vi "Wing.vi"() -> ()   [LabVIEW 2017]
doc: "This example performs writes and reads on a serial port, as directed by the user. You can press the Write and Read buttons, and change the Read Count, while the example is running.\n\nThe parameters set for the serial port must match the parameters of the connected instrument or device. In this example, the Read Count parameter specifies the number of bytes that the serial port reads. If there were more bytes at the port than the specified number, those bytes would not be read. If there were less bytes at the port than the specified number, you would receive a timeout error.\n\nThis example expands upon the flow control options for XON and XOFF, allowing the user to choose those control characters. Also, the user can enable or disable a termination character. Some devices require a termination character in order to identify the end of command strings. Some devices send a termination character to signify the end of data to be read. This example shows how you can end the Read operation once a termination character is detected in the buffer and/or append a termination character at the end of the Write data."
uses:
  subVIs/Serial - Settings.ctl
  subVIs/Serial - XON-XOFF Characters.ctl
  subVIs/Serial - ASCII Characters.ctl
  <vilib>/Analysis/baseanly.llb/Mean (DBL).vi
  <vilib>/DAQmx/read.llb/DAQmx Read (Analog 2D DBL NChan NSamp).vi
  <vilib>/Analysis/baseanly.llb/A x Vector.vi
  <vilib>/Instr/_visa.llb/VISA Configure Serial Port (Instr).vi
  <vilib>/DAQmx/create/channels.llb/DAQmx Create Channel (AI-Voltage-Basic).vi
  <vilib>/DAQmx/configure/timing.llb/DAQmx Timing (Sample Clock).vi
  <vilib>/express/express shared/transition.llb/Dynamic To Waveform Array.vi
  <vilib>/express/express arith-compare/Formula/Block/exnFormulaBlock how many pts in the wave.vi
  <vilib>/express/express shared/ex_Modify Signal Name.vi
  <vilib>/express/express shared/transition.llb/Waveform Array To Dynamic.vi
  <vilib>/DAQmx/miscellaneous.llb/DAQmx Fill In Error Info.vi
  <vilib>/express/express signal manip/GetorSetDDTAttributes/Set DDT Attributes/SetT0.vi
  <vilib>/express/express arith-compare/Formula/XNode/ExpressFormulaBlockNode.xnode
  <vilib>/express/express signal manip/GetorSetDDTAttributes/Set DDT Attributes/Set DDT Properties.xnode
  <vilib>/regexp/Match Regular Expression.xnode
  <vilib>/Analysis/NI_AALBase.lvlib
panel:
  out "New Bias Volt":dbl[][](array[numeric])
  out "New Bias Vec":dbl[](array[numeric])
  in  "Transform":T1
  in  "Tab Control":T2(tab)
  out "Drag (N)":dbl format="%#_3g"
  out "Lift (N)":dbl format="%#_3g"
  out "Calculated Density":dbl
  in  "Specific Gas Constant R":dbl
  in  "Ambient Temperature":dbl
  in  "Ambient Pressure":dbl
  out "Raw Voltage":dbl format="%#_4g"
  out "Airspeed":dbl
  out "Dynamic Pressure":dbl format="%#_4g"
  out "Transformed Lift and Drag Data":cluster{dbl, dbl}(graph)
  out "Position\n(relative to zeroed position)":dbl format="%#.3g"
  in  "Initiate Traverse&Log":bool
  in  "Stepper Control COM Port\n(changes require VI restart)":refnum<visa-resource-name>="COM1"
  out "Motion Status":string
  out "Controller Time":string
  out "Torque Units 2":string
  out "Force Units 2":string
  out "Measurement":dbl[][](graph) caption="Resolved Load Cell Data"
  in  "Bias":bool
  in  "Unbias":bool
  in  "Traverse Sweep":bool
  in  "Jog":bool
  in  "Jog Step (deg)":dbl
  in  "Zero":bool
  in  "Go Home":bool
  in  "Stop Motor":bool
  in  "Jog Mode":bool
  in  "1°":bool
  in  "0.25°":bool
  in  "-0.25°":bool
  in  "-1°":bool
  out "Factory-Calculated Calibration Matrix":dbl[][](array[numeric])
  out "Raw Strain Gauge Voltages":dbl[][](array[numeric]) format="%#_4g"
  out "Forces/Torques (X Y Z L M N) (N/Nm)":dbl[][](array[numeric]) format="%0.2f"
  out "Biased Voltages":dbl[](array[numeric]) format="%#.4g"
  out "RegEx 3":string
  out "whole match 3":string
  out "RegEx 2":string
  out "whole match 2":string
  out "whole match":string
  out "RegEx":string
  # "Data Collection"
  # "Wing Position Control"
  # "deg"
  # "Wind Speed Using Baratron"
  # "Air Density Calculation"
  # "1.016mmHg = 1 V"
  # "kPa"
  # "J/kgK"
  # "kg/m^3"
  # "C"
  # "Torr"
  # "m/s"
  # "Voltage to Load Conversions"
  # "-"
  # "="
  # "("
  # ")"
  # "x"
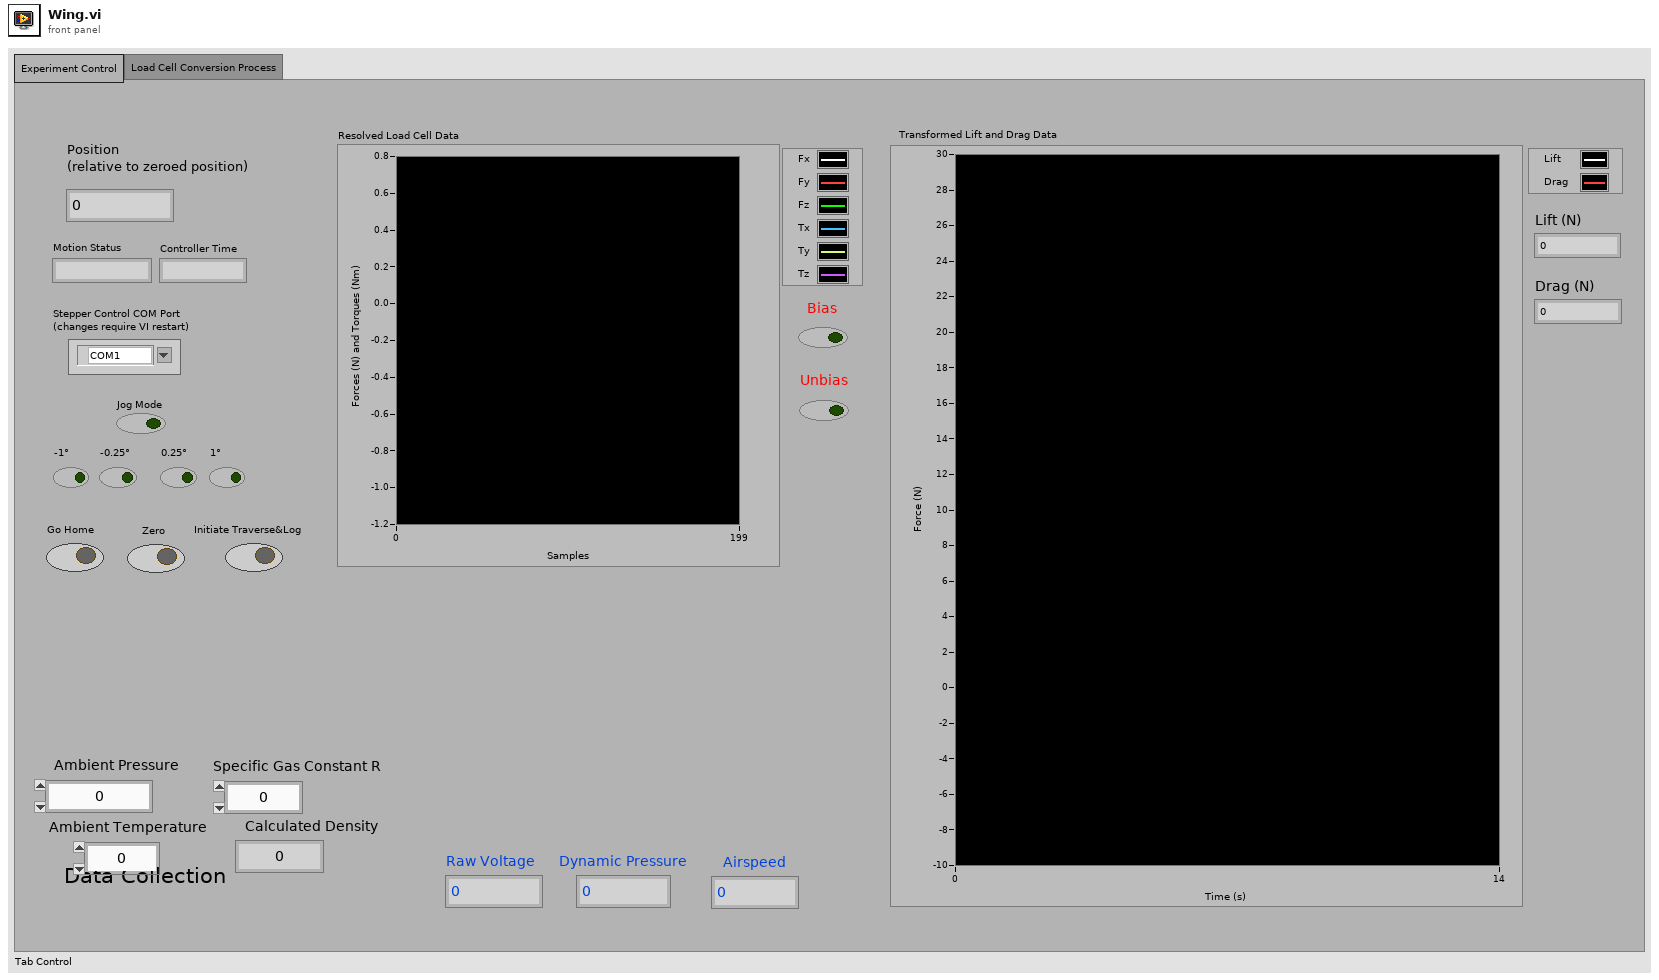
[diagram p1: front panel]
types:
  T1 = cluster{"Dx":dbl, "Dy":dbl, "Dz":dbl, "Rx":dbl, "Ry":dbl, "Rz":dbl}
  T2 = enum32{"Experiment Control", "Load Cell Conversion Process"}
  T3 = typedef "Serial - XON-XOFF Characters.ctl" = cluster{"XON":T4, "XOFF":T4}
  T4 = typedef "Serial - ASCII Characters.ctl" = enum16{"NUL", "SOH", "STX", "ETX", "EOT", "ENQ", "ACK", "BEL", "BS", "HT", "LF", "VT", "FF", "CR", "SO", "SI", "DLE", "DC1", "DC2", "DC3", "DC4", "NAK", "SYN", "ETB", "CAN", "EM", "SUB", "ESC", "FS", "GS", "RS", "US", "SP", "!", "\"", "#", "$", "%", "&", "'", "(", ")", "*", "+", ",", "- (-)", ".", "/", "0", "1", "2", "3", "4", "5", "6", "7", "8", "9", ":", ";", "<", "=", ">", "?", "@", "A", "B", "C", "D", "E", "F", "G", "H", "I", "J", "K", "L", "M", "N", "O", "P", "Q", "R", "S", "T", "U", "V", "W", "X", "Y", "Z", "[", "\\", "]", "^", "_", "`", "a", "b", "c", "d", "e", "f", "g", "h", "i", "j", "k", "l", "m", "n", "o", "p", "q", "r", "s", "t", "u", "v", "w", "x", "y", "z", "{", "|", "}", "~"}
  T5 = typedef "Serial - Settings.ctl" = cluster{"baud rate":u32, "data bits":u16, "parity":enum16{"None", "Odd", "Even", "Mark", "Space"}, "stop bits":u16, "flow control":u16}
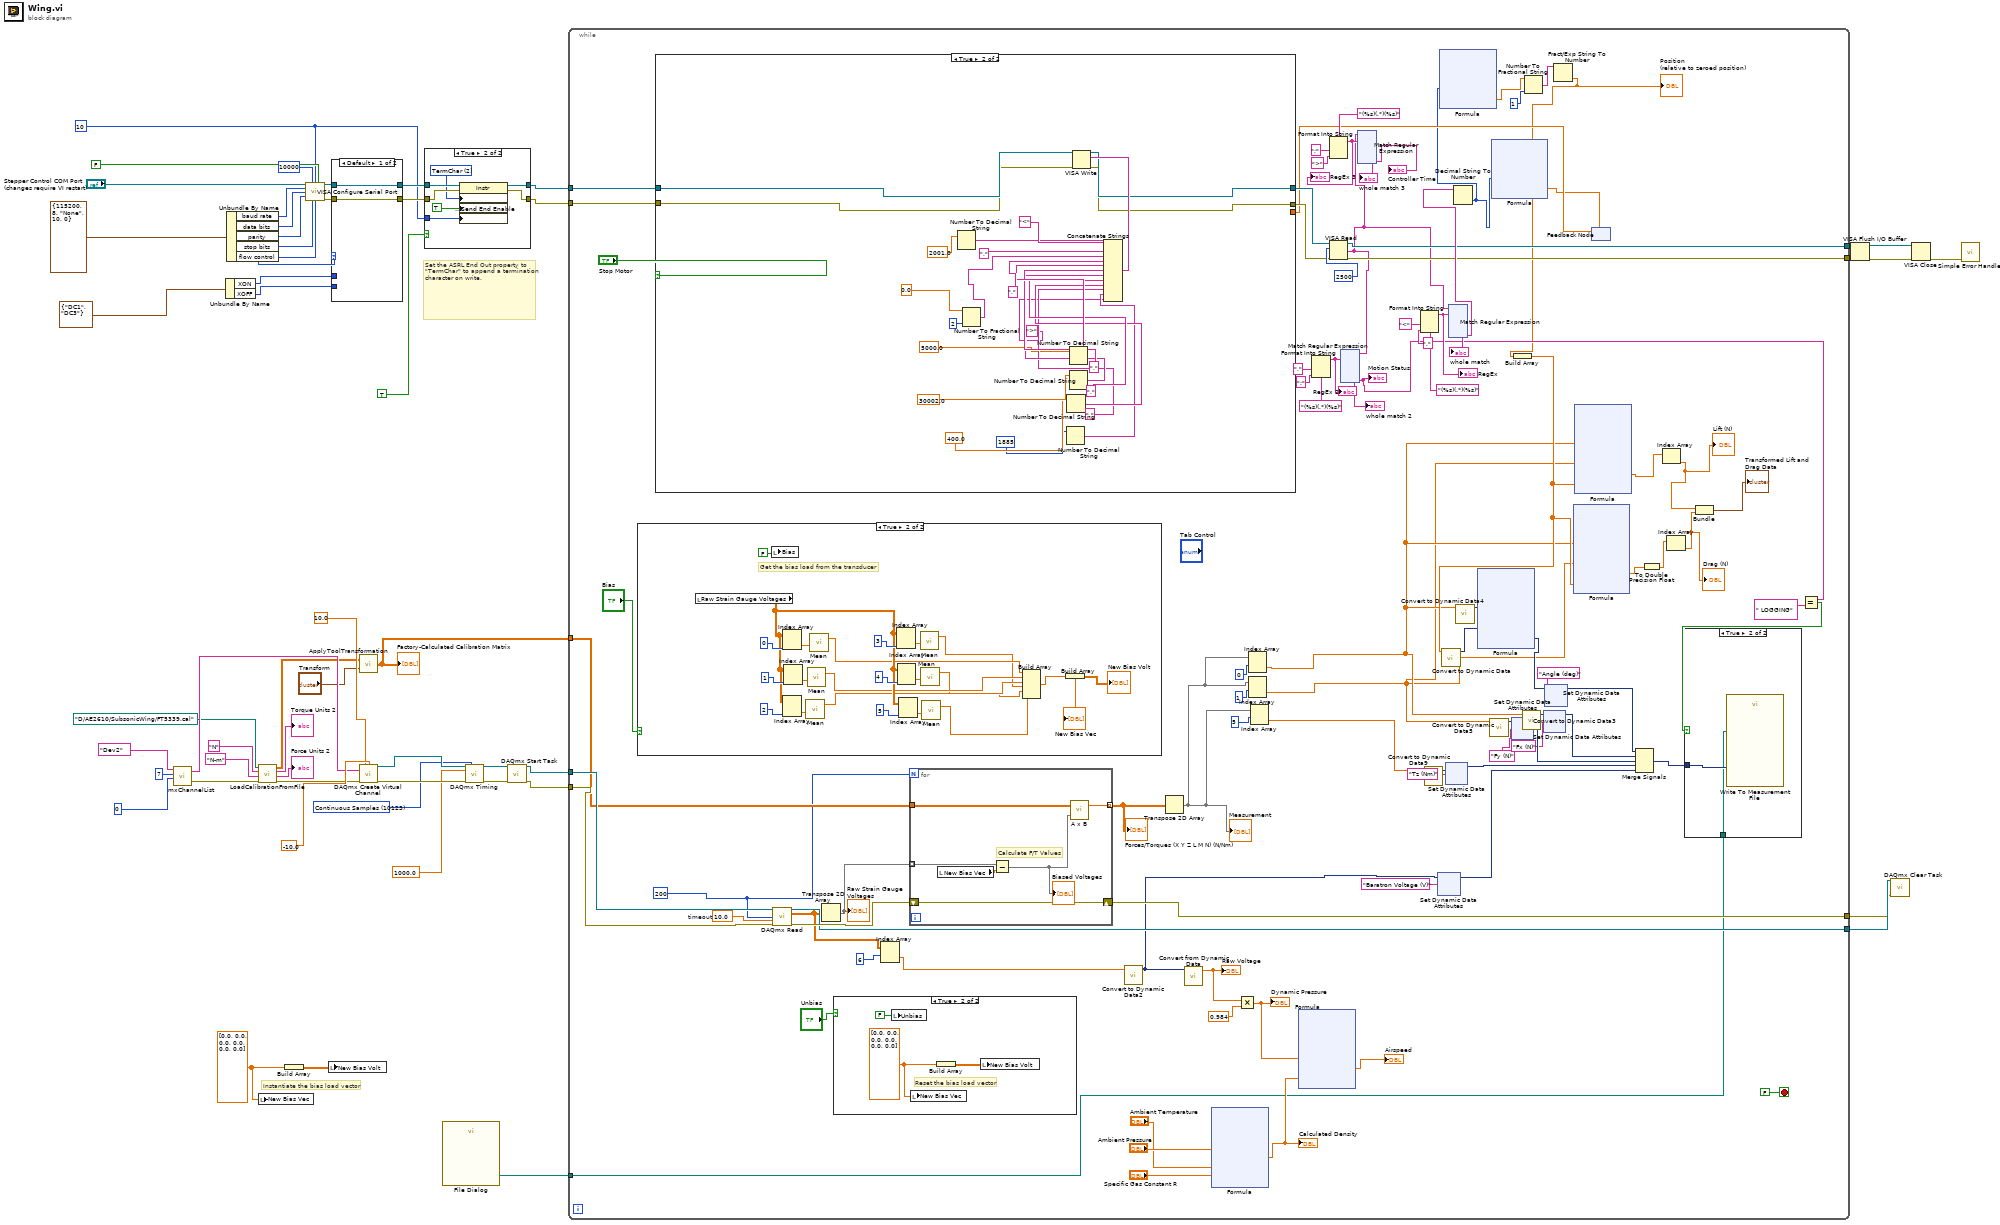
[diagram p0: block diagram]
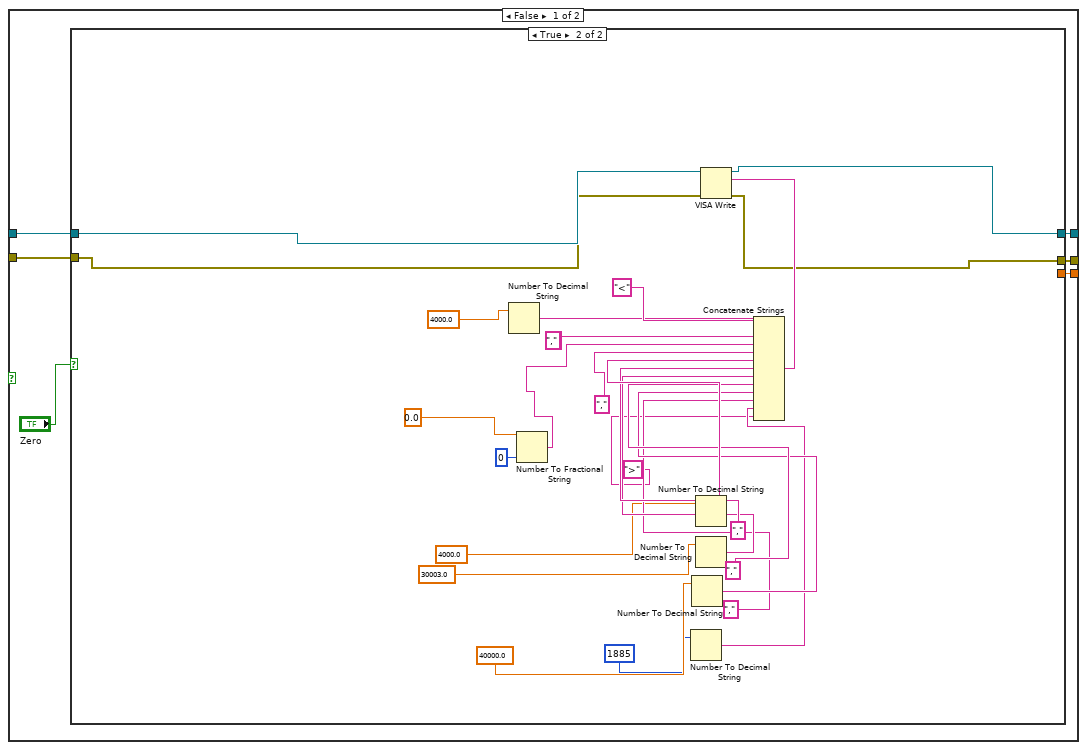
[diagram p5: hidden frame]
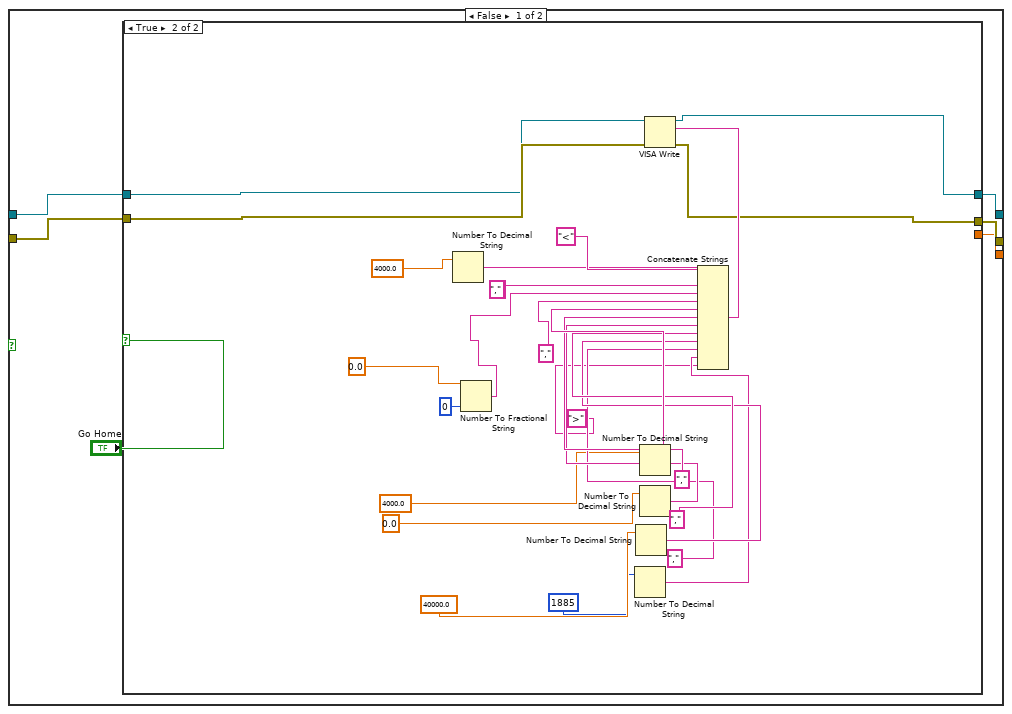
[diagram p6: hidden frame]
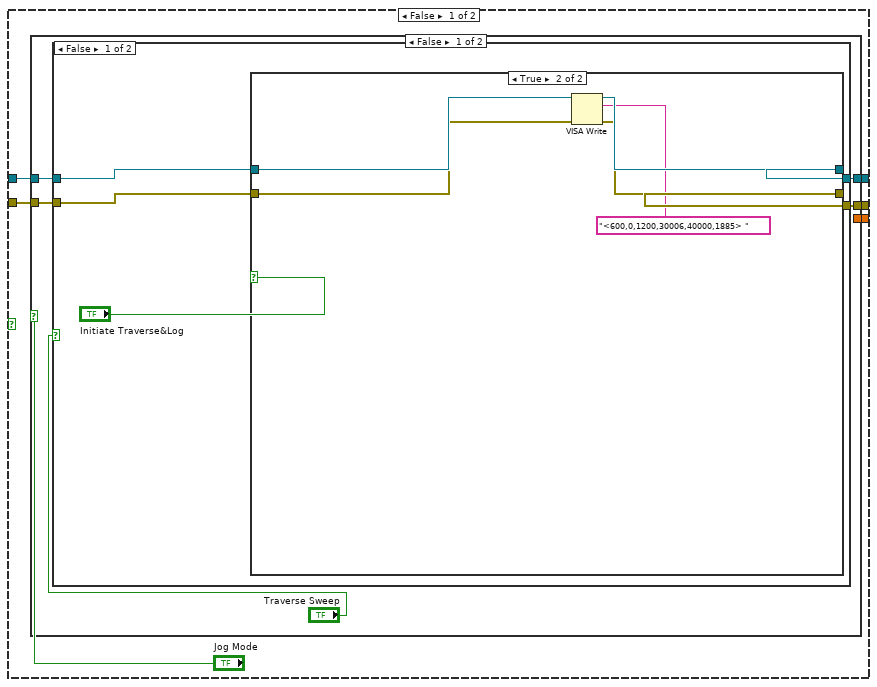
[diagram p7: hidden frame]
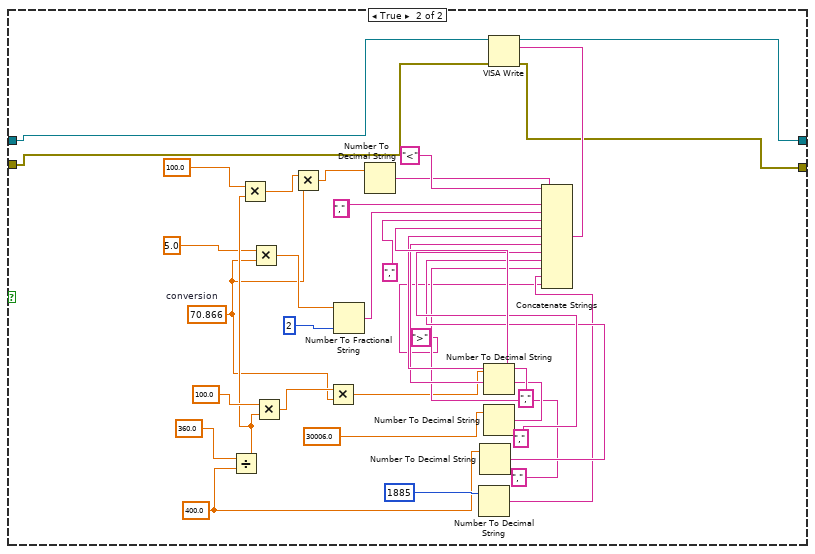
[diagram p9: hidden frame]
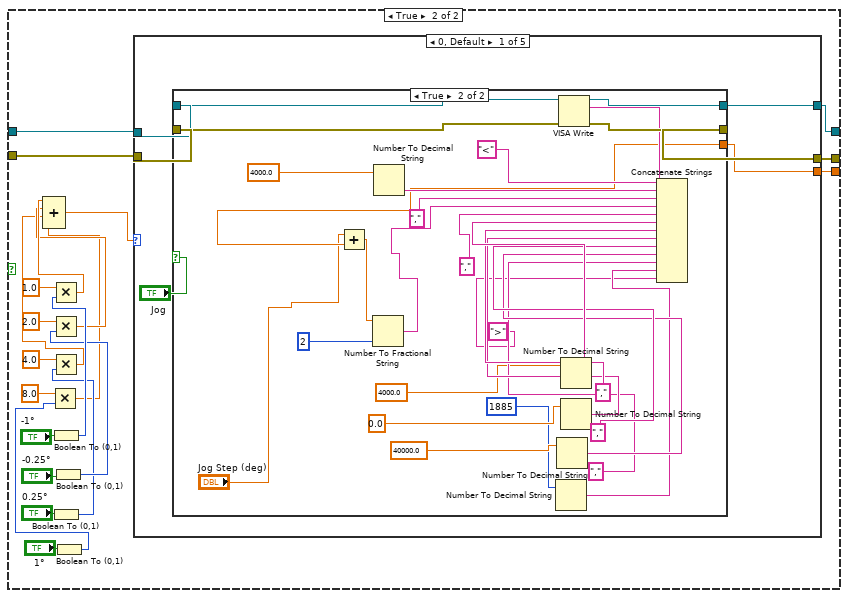
[diagram p10: hidden frame]
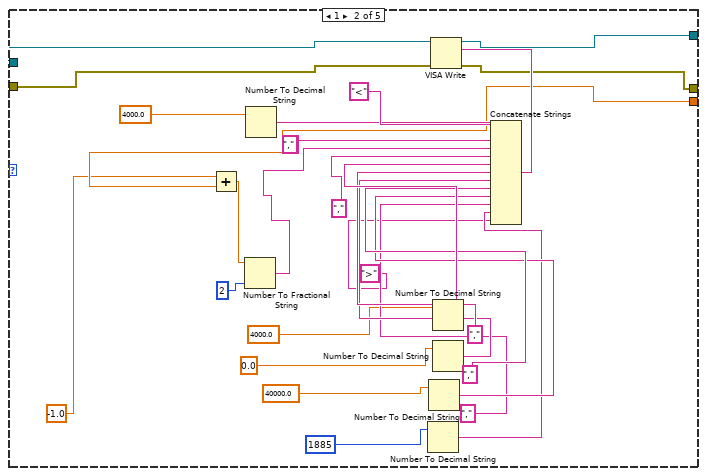
[diagram p12: hidden frame]
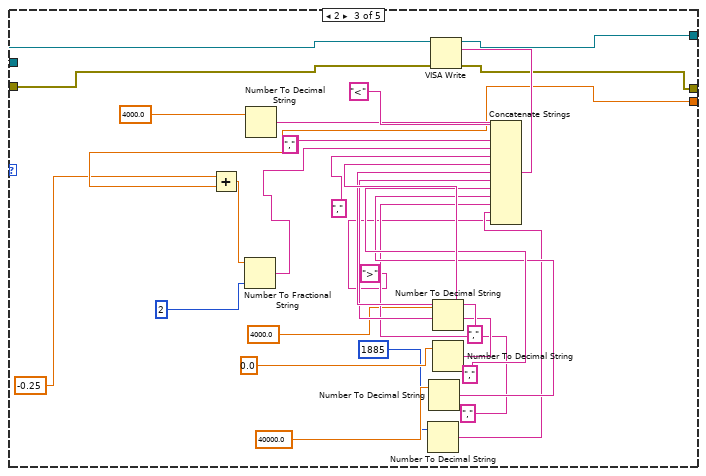
[diagram p13: hidden frame]
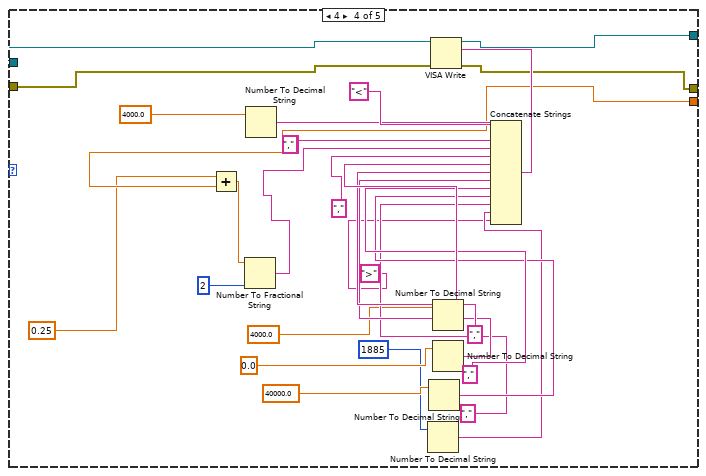
[diagram p14: hidden frame]
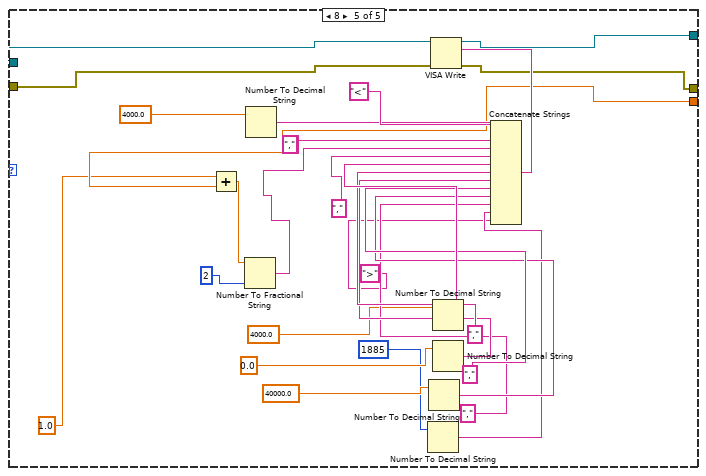
[diagram p15: hidden frame]
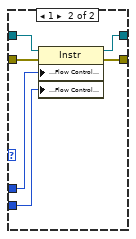
[diagram p17: hidden frame]
diagram:
  w2 = dbl[] [0.0, 0.0, 0.0, 0.0, 0.0, 0.0]
  w25 = 10123 items=["Finite Samples"=10178, "Continuous Samples"=10123] ("sample mode")
  w37 = u8 10 ("Termination Character")
  # "Instantiate the bias load vector"
  # "Set the ASRL End Out property to \"TermChar\" to append a termination character on write."
  n1 = call "mxChannelList.vi"("First Channel"=i16 0, "Number of Channels"=7, "DAQmx Device Name"=tag "Dev2" ("DAQ Card")) -> ("error out"=w10:errorcluster, "Channel List"=w19:string)  [unwired: 1 in]
  n2 = Unbundle By Name(T3 {"XON"=enum."DC1", "XOFF"=enum."DC3"} ("XON/XOFF Characters")) -> ("XON"=w42:T4, "XOFF"=w41:T4)
  n3 = Unbundle By Name(T5 {"baud rate"=115200, "data bits"=8, "parity"=enum."None", "stop bits"=10, "flow control"=0} ("Serial Settings")) -> ("baud rate"=w47:u32, "data bits"=w48:u16, "parity"=w49:enum16{"None", "Odd", "Even", "Mark", "Space"}, "stop bits"=w50:u16, "flow control"=w43:u16)
  n4 = call "LoadCalibrationFromFile.vi"("Error In"=w10, "User Torque Units"="N-m" ("Torque Units"), "User Force Units"="N" ("Force Units"), "Cal File Path"=path "D:/AE2610/SubsonicWing/FT5339.cal" ("Calibration File")) -> ("Error Out"=w9:errorcluster, "Calibration Force Units"=→"Force Units 2":string, "Calibration Torque Units"=→"Torque Units 2":string, "Calibration Matrix"=w15:dbl[][])
  n5 = local write "New Bias Vec"(w2) -> ()
  n6 = Build Array(w2) -> (w1:dbl[][])
  n7 = call-poly "VISA Configure Serial Port"("VISA resource name"="Stepper Control COM Port\n(changes require VI restart)", "timeout (10sec)"=u32 10000, "termination char\n(0xA = '\\n' = LF)"=w37, "Enable Termination\nChar (T)"=FALSE ("End Read on Termination Character?"), "baud rate (9600)"=w47, "data bits (8)"=w48, "parity (0:none)"=w49, "stop bits (10: 1 bit)"=w50, "flow control (0:none)"=w43) -> ("VISA resource name out"=w51:refnum<visa-resource-name>, "error out"=w52:errorcluster)  [unwired: 1 in, 4 out]
  n8 = local write "New Bias Volt"(w1) -> ()
  n9 = case shown="Default" w43 {
    tunnel: [w55 w62] -> w40
    tunnel: [w56 w61] -> w39
    tunnel: w52 -> [w55 w60]
    tunnel: w51 -> [w56 w59]
    tunnel: w42 -> [_ w58]
    tunnel: w41 -> [_ w57]
    frame Default {
    }
    frame 1 {
      n10 = property class="Instr"(reference=w59, error in=w60, "Serial Settings:Flow Control XON Character"=w58, "Serial Settings:Flow Control XOFF Character"=w57) -> (reference out=w61:refnum<visa-resource-name>, error out=w62:errorcluster)
    }
  }
  n11 = call "ApplyToolTransformation.vi"("Transform"="Transform", "Calibration Matrix"=w15) -> ("Transformed Calibration Matrix"=w6:dbl[][])
  "Factory-Calculated Calibration Matrix" <- w6
  n12 = call-poly <vilib>:"DAQmx Create Virtual Channel.vi"("maximum value"=10.0 ("Maximum Value"), "minimum value"=-10.0 ("Minimum Value"), "physical channels"=w19, "error in"=w9) -> ("task out"=w26:refnum<k21>, "error out"=w27:errorcluster)  [unwired: 10 in]
  n13 = case shown="True" TRUE ("End Write on Termination Character?") {
    tunnel: w39 -> [w63 w71]
    tunnel: w40 -> [w64 w70]
    tunnel: [w63 w69] -> w36
    tunnel: [w64 w68] -> w35
    tunnel: w37 -> [_ w66]
    frame False {
    }
    frame True {
      w67 = u16 2 items=["None", "LastBit", "TermChar", "Break"] ("Serial Settings:Serial End Mode for Writes")
      n14 = property class="Instr"(reference=w71, error in=w70, "Serial Settings:End Mode for Writes"=w67, "Message Based Settings:Send End Enable"=TRUE, "Message Based Settings:Termination Character"=w66) -> (reference out=w69:refnum<visa-resource-name>, error out=w68:errorcluster)
    }
  }
  n15 = call "File Dialog"() -> ("selected path"=w3:path)  [unwired: 12 in, 3 out]
  n16 = call-poly <vilib>:"DAQmx Timing.vi"("task/channels in"=w26, "sample mode"=w25, "rate"=1000.0 ("Sample Rate"), "error in"=w27) -> ("task out"=w24:refnum<k21>, "error out"=w18:errorcluster)  [unwired: 10 in]
  n17 = call <vilib>:"DAQmx Start Task.vi"("task/channels in"=w24, "error in"=w18) -> ("task out"=w8:refnum<k21>, "error out"=w7:errorcluster)  [unwired: 12 in]
  n18 = while {
    tunnel: w36 -> [w149]
    tunnel: w35 -> [w148]
    tunnel: [w147] -> w33
    tunnel: [w146] -> w34
    tunnel: w8 -> [w133]
    tunnel: w7 -> [w132]
    tunnel: w6 -> [w129]
    tunnel: [w127] -> w5
    tunnel: [w124] -> w4
    tunnel: w3 -> [w85]
    stop <- FALSE stop-if-true
    w128 = 200 ("Samples to Read")
    w134 = 10.0  # timeout
    n19 = case shown="True" "Bias" {
      frame False {
      }
      frame True {
        # "Get the bias load from the transducer"
        n20 = local read "Raw Strain Gauge Voltages"() -> (w705:dbl[][])
        n21 = local write "Bias"(FALSE) -> ()
        n22 = Index Array(array=w705, index (col)=0 ("disabled index (col)")) -> (element=w718:dbl[])  [unwired: 1 in]
        n23 = Index Array(array=w705, index (col)=2 ("disabled index (col)")) -> (element=w713:dbl[])  [unwired: 1 in]
        n24 = Index Array(array=w705, index (col)=1 ("disabled index (col)")) -> (element=w715:dbl[])  [unwired: 1 in]
        n25 = call-poly <vilib>:"Mean.vi"("X"=w713) -> ("mean"=w702:dbl)  [unwired: 1 out]
        n26 = call-poly <vilib>:"Mean.vi"("X"=w715) -> ("mean"=w703:dbl)  [unwired: 1 out]
        n27 = call-poly <vilib>:"Mean.vi"("X"=w718) -> ("mean"=w704:dbl)  [unwired: 1 out]
        n28 = Index Array(array=w705, index (col)=3 ("disabled index (col)")) -> (element=w711:dbl[])  [unwired: 1 in]
        n29 = Index Array(array=w705, index (col)=4 ("disabled index (col)")) -> (element=w709:dbl[])  [unwired: 1 in]
        n30 = Index Array(array=w705, index (col)=5 ("disabled index (col)")) -> (element=w707:dbl[])  [unwired: 1 in]
        n31 = call-poly <vilib>:"Mean.vi"("X"=w711) -> ("mean"=w701:dbl)  [unwired: 1 out]
        n32 = call-poly <vilib>:"Mean.vi"("X"=w709) -> ("mean"=w700:dbl)  [unwired: 1 out]
        n33 = call-poly <vilib>:"Mean.vi"("X"=w707) -> ("mean"=w699:dbl)  [unwired: 1 out]
        n34 = Build Array(w704, w703, w702, w701, w700, w699) -> (w698:dbl[])
        "New Bias Vec" <- w698
        n35 = Build Array(w698) -> (→"New Bias Volt":dbl[][])
      }
    }
    n36 = call-poly <vilib>:"DAQmx Read.vi"("task/channels in"=w133, "number of samples per channel"=w128, "timeout"=w134, "error in"=w132) -> ("task out"=w127:refnum<k21>, "data"=w96:dbl[][], "error out"=w131:errorcluster)  [unwired: 9 in]
    n37 = Transpose 2D Array(2D array=w96) -> (transposed array=w130:dbl[][])
    "Raw Strain Gauge Voltages" <- w130
    n38 = case shown="True" "Unbias" {
      frame False {
      }
      frame True {
        w695 = dbl[] [0.0, 0.0, 0.0, 0.0, 0.0, 0.0]
        # "Reset the bias load vector"
        n39 = local write "Unbias"(FALSE) -> ()
        n40 = local write "New Bias Vec"(w695) -> ()
        n41 = Build Array(w695) -> (w694:dbl[][])
        n42 = local write "New Bias Volt"(w694) -> ()
      }
    }
    n43 = Index Array(array=w96, index (row)=6) -> (element=w94:dbl[])  [unwired: 1 in]
    n44 = for {
      N: w128 -> [_]
      tunnel: [w722] -> w120 mode=indexing
      shift-right: [w721] -> w124
      shift-left: w131 -> [w721]
      tunnel: w130 -> [w724] mode=indexing
      tunnel: w129 -> [w720]
      # "Calculate F/T Values"
      n45 = local read "New Bias Vec"() -> (w723:dbl[])
      n46 = Subtract(x=w724, y=w723) -> (x-y=w719:dbl[])
      "Biased Voltages" <- w719
      n47 = call-poly <vilib>:"A x B.vi"("Vector"=w719, "A"=w720) -> ("A x Vector"=w722:dbl[])  [unwired: 1 out]
    }
    "Forces/Torques (X Y Z L M N) (N/Nm)" <- w120
    n48 = call "Convert to Dynamic Data2"("Array"=w94) -> ("Dynamic Data Type"=w76:dynamicdata)  [unwired: 3 in]
    n49 = Transpose 2D Array(2D array=w120) -> (transposed array=w119:dbl[][])
    "Measurement" <- w119
    n50 = call "Convert from Dynamic Data"("Dynamic Data Type"=w76) -> ("Scalar"=w91:dbl)  [unwired: 3 in]
    "Raw Voltage" <- w91
    n51 = xnode "Formula"("P"="Ambient Pressure", "T"="Ambient Temperature", "R"="Specific Gas Constant R") -> ("Result"=w87:dbl)  [unwired: 1 in, 1 out]
    "Calculated Density" <- w87
    n52 = Multiply(x=w91, y=0.984) -> (x*y=w84:dbl)
    "Dynamic Pressure" <- w84
    n53 = Index Array(array=w119, index (row)=0 ("index")) -> (element=w83:dbl[])  [unwired: 1 in]
    n54 = Index Array(array=w119, index (row)=1 ("index")) -> (element=w80:dbl[])  [unwired: 1 in]
    n55 = Index Array(array=w119, index (row)=5 ("index")) -> (element=w78:dbl[])  [unwired: 1 in]
    n56 = xnode "Formula"("del P"=w84, "Density"=w87) -> ("Result"=→"Airspeed":dbl)  [unwired: 1 in, 1 out]
    n57 = Format Into String(format string="(%s)(.*)(%s)", "," ("WordBefore"), ";" ("WordAfter")) -> (resulting string=w163:string)  [unwired: 2 in, 1 out]
    "RegEx 2" <- w163
    n58 = Format Into String(format string="(%s)(.*)(%s)", ";" ("WordBefore"), ">" ("WordAfter")) -> (resulting string=w145:string)  [unwired: 2 in, 1 out]
    "RegEx 3" <- w145
    n59 = Format Into String(format string="(%s)(.*)(%s)", "<" ("WordBefore"), "," ("WordAfter")) -> (resulting string=w160:string)  [unwired: 2 in, 1 out]
    "RegEx" <- w160
    n60 = call "Convert to Dynamic Data9"("Array"=w78) -> ("Dynamic Data Type"=w77:dynamicdata)  [unwired: 3 in]
    n61 = xnode ("Set Dynamic Data Attributes")("Signals In"=w76, "Signal Name"="Baratron Voltage (V)") -> ("Signals Out"=w74:dynamicdata)  [unwired: 2 in, 1 out]
    n62 = xnode ("Set Dynamic Data Attributes")("Signals In"=w77, "Signal Name"="Tz (Nm)") -> ("Signals Out"=w75:dynamicdata)  [unwired: 2 in, 1 out]
    n63 = call "Convert to Dynamic Data4"("Array"=w83) -> ("Dynamic Data Type"=w81:dynamicdata)  [unwired: 3 in]
    n64 = call "Convert to Dynamic Data5"("Array"=w80) -> ("Dynamic Data Type"=w79:dynamicdata)  [unwired: 3 in]
    n65 = xnode ("Set Dynamic Data Attributes")("Signals In"=w79, "Signal Name"="Fy (N)") -> ("Signals Out"=w114:dynamicdata)  [unwired: 2 in, 1 out]
    n66 = call "Convert to Dynamic Data3"("Array"=w83) -> ("Dynamic Data Type"=w82:dynamicdata)  [unwired: 3 in]
    n67 = xnode ("Set Dynamic Data Attributes")("Signals In"=w82, "Signal Name"="Fx (N)") -> ("Signals Out"=w115:dynamicdata)  [unwired: 2 in, 1 out]
    n68 = feedback #1() -> (w137:dbl)  [unwired: 1 in]
    n69 = case shown="True" "Stop Motor" {
      tunnel: [w738 w1016] -> w157
      tunnel: [w737 w1017] -> w156
      tunnel: w149 -> [w736 w1019]
      tunnel: w148 -> [w735 w1018]
      tunnel: w137 -> [w734 _]
      frame False {
        n70 = case shown="True" "Zero" {
          tunnel: [w744 w991] -> w738
          tunnel: [w743 w992] -> w737
          tunnel: w736 -> [w742 w994]
          tunnel: w735 -> [w741 w993]
          tunnel: w734 -> [w740 _]
          frame False {
            n71 = case shown="True" "Go Home" {
              tunnel: [w750 w966] -> w744
              tunnel: [w749 w967] -> w743
              tunnel: w742 -> [w748 w968]
              tunnel: w741 -> [w747 w969]
              tunnel: w740 -> [w745 _]
              frame False {
                n72 = case shown="False" "Jog Mode" {
                  tunnel: [w755 w818] -> w750
                  tunnel: [w754 w819] -> w749
                  tunnel: w748 -> [w753 w822]
                  tunnel: w747 -> [w752 w821]
                  tunnel: w745 -> [_ w820]
                  frame False {
                    n73 = case shown="False" "Traverse Sweep" {
                      tunnel: [w759 w769] -> w755
                      tunnel: [w758 w768] -> w754
                      tunnel: w753 -> [w757 w771]
                      tunnel: w752 -> [w756 w770]
                      frame False {
                        n74 = case shown="True" "Initiate Traverse&Log" {
                          tunnel: w757 -> [w762 w767]
                          tunnel: w756 -> [w761 w766]
                          tunnel: [w762 w765] -> w758
                          tunnel: [w761 w764] -> w759
                          frame False {
                          }
                          frame True {
                            n75 = VISA Write(VISA resource name=w767, write buffer="<600,0,1200,30006,40000,1885> ", error in (no error)=w766) -> (VISA resource name out=w765:refnum<visa-resource-name>, error out=w764:errorcluster)  [unwired: 1 out]
                          }
                        }
                      }
                      frame True {
                        w783 = 400.0 ("Steps/rev 2")
                        w772 = 70.866  # conversion
                        (unwired) ","
                        n76 = Divide(x=360.0, y=w783) -> (x/y=w779:dbl)
                        n77 = Multiply(x=100.0 ("Acceleration (mm/s^2) 2"), y=w779) -> (x*y=w774:dbl)
                        n78 = Multiply(x=5.0 ("Position (mm) 2"), y=w772) -> (x*y=w778:dbl)
                        n79 = Multiply(x=100.0 ("Velocity (mm/s) 2"), y=w779) -> (x*y=w776:dbl)
                        n80 = Multiply(x=w774, y=w772) -> (x*y=w773:dbl)
                        n81 = Multiply(x=w776, y=w772) -> (x*y=w775:dbl)
                        n82 = Number To Fractional String(number=w778, precision (6)=i16 2) -> (F-format string=w785:string)  [unwired: 2 in]
                        n83 = Number To Decimal String(number=w773) -> (decimal integer string=w797:string)  [unwired: 1 in]
                        n84 = Number To Decimal String(number=1885 ("Password 2")) -> (decimal integer string=w788:string)  [unwired: 1 in]
                        n85 = Number To Decimal String(number=w783) -> (decimal integer string=w790:string)  [unwired: 1 in]
                        n86 = Number To Decimal String(number=w775) -> (decimal integer string=w794:string)  [unwired: 1 in]
                        n87 = Number To Decimal String(number=30006.0 ("Number of Bounces 2")) -> (decimal integer string=w792:string)  [unwired: 1 in]
                        n88 = Concatenate Strings("<", w797, ",", w785, ",", w794, ",", w792, ",", w790, ",", w788, ">") -> (w786:string)
                        n89 = VISA Write(VISA resource name=w771, write buffer=w786, error in (no error)=w770) -> (VISA resource name out=w768:refnum<visa-resource-name>, error out=w769:errorcluster)  [unwired: 1 out]
                      }
                    }
                  }
                  frame True {
                    n90 = Boolean To (0,1)(Boolean="-1°") -> (0, 1=w809:i16)
                    n91 = Multiply(x=1.0, y=w809) -> (x*y=w805:dbl)
                    n92 = Boolean To (0,1)(Boolean="0.25°") -> (0, 1=w807:i16)
                    n93 = Multiply(x=4.0, y=w807) -> (x*y=w803:dbl)
                    n94 = Boolean To (0,1)(Boolean="-0.25°") -> (0, 1=w808:i16)
                    n95 = Multiply(x=2.0, y=w808) -> (x*y=w804:dbl)
                    n96 = Boolean To (0,1)(Boolean="1°") -> (0, 1=w806:i16)
                    n97 = Multiply(x=8.0, y=w806) -> (x*y=w802:dbl)
                    n98 = Compound Arithmetic op=ADD(w805, w804, w803, w802) -> (w801:dbl)
                    n99 = case shown="0, Default" w801 {
                      tunnel: w822 -> [w826 w860 w888 w915 w942]
                      tunnel: w821 -> [w827 w861 w889 w916 w943]
                      tunnel: w820 -> [w823 w859 w887 w914 w941]
                      tunnel: [w825 w863 w891 w918 w945] -> w819
                      tunnel: [w824 w862 w890 w917 w944] -> w818
                      frame 0, Default {
                        n100 = case shown="True" "Jog" {
                          tunnel: w826 -> [w830 w857]
                          tunnel: w827 -> [w829 w856]
                          tunnel: [w830 w855] -> w825
                          tunnel: [w829 w854] -> w824
                          tunnel: w823 -> [_ w833]
                          frame False {
                          }
                          frame True {
                            n101 = Add(x="Jog Step (deg)", y=w833) -> (x+y=w832:dbl)
                            n102 = Number To Fractional String(number=w832, precision (6)=i16 2) -> (F-format string=w835:string)  [unwired: 2 in]
                            n103 = Number To Decimal String(number=4000.0 ("Acceleration (steps/s) 2")) -> (decimal integer string=w848:string)  [unwired: 1 in]
                            n104 = Number To Decimal String(number=1885 ("Password 2")) -> (decimal integer string=w839:string)  [unwired: 1 in]
                            n105 = Number To Decimal String(number=40000.0 ("Steps/rev 2")) -> (decimal integer string=w841:string)  [unwired: 1 in]
                            n106 = Number To Decimal String(number=4000.0 ("Velocity (steps/s) 2")) -> (decimal integer string=w845:string)  [unwired: 1 in]
                            n107 = Number To Decimal String(number=0.0 ("Number of Bounces 2")) -> (decimal integer string=w843:string)  [unwired: 1 in]
                            n108 = Concatenate Strings("<", w848, ",", w835, ",", w845, ",", w843, ",", w841, ",", w839, ">") -> (w837:string)
                            n109 = VISA Write(VISA resource name=w857, write buffer=w837, error in (no error)=w856) -> (VISA resource name out=w855:refnum<visa-resource-name>, error out=w854:errorcluster)  [unwired: 1 out]
                          }
                        }
                      }
                      frame 1 {
                        (unwired) ","
                        n110 = Add(x=-1.0 ("Jog Step (angle) 2"), y=w859) -> (x+y=w864:dbl)
                        n111 = Number To Fractional String(number=w864, precision (6)=i16 2) -> (F-format string=w866:string)  [unwired: 2 in]
                        n112 = Number To Decimal String(number=4000.0 ("Acceleration (steps/s) 2")) -> (decimal integer string=w879:string)  [unwired: 1 in]
                        n113 = Number To Decimal String(number=1885 ("Password 3")) -> (decimal integer string=w870:string)  [unwired: 1 in]
                        n114 = Number To Decimal String(number=40000.0 ("Steps/rev 3")) -> (decimal integer string=w872:string)  [unwired: 1 in]
                        n115 = Number To Decimal String(number=4000.0 ("Velocity (steps/s) 2")) -> (decimal integer string=w876:string)  [unwired: 1 in]
                        n116 = Number To Decimal String(number=0.0 ("Number of Bounces 2")) -> (decimal integer string=w874:string)  [unwired: 1 in]
                        n117 = Concatenate Strings("<", w879, ",", w866, ",", w876, ",", w874, ",", w872, ",", w870, ">") -> (w868:string)
                        n118 = VISA Write(VISA resource name=w860, write buffer=w868, error in (no error)=w861) -> (VISA resource name out=w863:refnum<visa-resource-name>, error out=w862:errorcluster)  [unwired: 1 out]
                      }
                      frame 2 {
                        (unwired) ","
                        n119 = Add(x=-0.25 ("Jog Step (angle) 2"), y=w887) -> (x+y=w892:dbl)
                        n120 = Number To Fractional String(number=w892, precision (6)=i16 2) -> (F-format string=w893:string)  [unwired: 2 in]
                        n121 = Number To Decimal String(number=4000.0 ("Acceleration (steps/s) 2")) -> (decimal integer string=w906:string)  [unwired: 1 in]
                        n122 = Number To Decimal String(number=1885 ("Password 4")) -> (decimal integer string=w897:string)  [unwired: 1 in]
                        n123 = Number To Decimal String(number=40000.0 ("Steps/rev 4")) -> (decimal integer string=w899:string)  [unwired: 1 in]
                        n124 = Number To Decimal String(number=4000.0 ("Velocity (steps/s) 2")) -> (decimal integer string=w903:string)  [unwired: 1 in]
                        n125 = Number To Decimal String(number=0.0 ("Number of Bounces 2")) -> (decimal integer string=w901:string)  [unwired: 1 in]
                        n126 = Concatenate Strings("<", w906, ",", w893, ",", w903, ",", w901, ",", w899, ",", w897, ">") -> (w895:string)
                        n127 = VISA Write(VISA resource name=w888, write buffer=w895, error in (no error)=w889) -> (VISA resource name out=w891:refnum<visa-resource-name>, error out=w890:errorcluster)  [unwired: 1 out]
                      }
                      frame 4 {
                        (unwired) ","
                        n128 = Add(x=0.25 ("Jog Step (angle) 2"), y=w914) -> (x+y=w919:dbl)
                        n129 = Number To Fractional String(number=w919, precision (6)=i16 2) -> (F-format string=w920:string)  [unwired: 2 in]
                        n130 = Number To Decimal String(number=4000.0 ("Acceleration (steps/s) 2")) -> (decimal integer string=w933:string)  [unwired: 1 in]
                        n131 = Number To Decimal String(number=1885 ("Password 5")) -> (decimal integer string=w924:string)  [unwired: 1 in]
                        n132 = Number To Decimal String(number=40000.0 ("Steps/rev 5")) -> (decimal integer string=w926:string)  [unwired: 1 in]
                        n133 = Number To Decimal String(number=4000.0 ("Velocity (steps/s) 2")) -> (decimal integer string=w930:string)  [unwired: 1 in]
                        n134 = Number To Decimal String(number=0.0 ("Number of Bounces 2")) -> (decimal integer string=w928:string)  [unwired: 1 in]
                        n135 = Concatenate Strings("<", w933, ",", w920, ",", w930, ",", w928, ",", w926, ",", w924, ">") -> (w922:string)
                        n136 = VISA Write(VISA resource name=w915, write buffer=w922, error in (no error)=w916) -> (VISA resource name out=w918:refnum<visa-resource-name>, error out=w917:errorcluster)  [unwired: 1 out]
                      }
                      frame 8 {
                        (unwired) ","
                        n137 = Add(x=1.0 ("Jog Step (angle) 2"), y=w941) -> (x+y=w946:dbl)
                        n138 = Number To Fractional String(number=w946, precision (6)=i16 2) -> (F-format string=w947:string)  [unwired: 2 in]
                        n139 = Number To Decimal String(number=4000.0 ("Acceleration (steps/s) 2")) -> (decimal integer string=w960:string)  [unwired: 1 in]
                        n140 = Number To Decimal String(number=1885 ("Password 6")) -> (decimal integer string=w951:string)  [unwired: 1 in]
                        n141 = Number To Decimal String(number=40000.0 ("Steps/rev 6")) -> (decimal integer string=w953:string)  [unwired: 1 in]
                        n142 = Number To Decimal String(number=4000.0 ("Velocity (steps/s) 2")) -> (decimal integer string=w957:string)  [unwired: 1 in]
                        n143 = Number To Decimal String(number=0.0 ("Number of Bounces 2")) -> (decimal integer string=w955:string)  [unwired: 1 in]
                        n144 = Concatenate Strings("<", w960, ",", w947, ",", w957, ",", w955, ",", w953, ",", w951, ">") -> (w949:string)
                        n145 = VISA Write(VISA resource name=w942, write buffer=w949, error in (no error)=w943) -> (VISA resource name out=w945:refnum<visa-resource-name>, error out=w944:errorcluster)  [unwired: 1 out]
                      }
                    }
                  }
                }
              }
              frame True {
                (unwired) ","
                n146 = Number To Decimal String(number=4000.0 ("Acceleration (steps/s) 3")) -> (decimal integer string=w985:string)  [unwired: 1 in]
                n147 = Number To Fractional String(number=0.0 ("Position (degrees) 3"), precision (6)=i16 0) -> (F-format string=w971:string)  [unwired: 2 in]
                n148 = Number To Decimal String(number=1885 ("Password 4")) -> (decimal integer string=w976:string)  [unwired: 1 in]
                n149 = Number To Decimal String(number=40000.0 ("Steps/rev 4")) -> (decimal integer string=w978:string)  [unwired: 1 in]
                n150 = Number To Decimal String(number=4000.0 ("Velocity (steps/s) 3")) -> (decimal integer string=w982:string)  [unwired: 1 in]
                n151 = Number To Decimal String(number=0.0 ("Number of Bounces 2")) -> (decimal integer string=w980:string)  [unwired: 1 in]
                n152 = Concatenate Strings("<", w985, ",", w971, ",", w982, ",", w980, ",", w978, ",", w976, ">") -> (w974:string)
                n153 = VISA Write(VISA resource name=w968, write buffer=w974, error in (no error)=w969) -> (VISA resource name out=w967:refnum<visa-resource-name>, error out=w966:errorcluster)  [unwired: 1 out]
              }
            }
          }
          frame True {
            (unwired) ","
            n154 = Number To Decimal String(number=4000.0 ("Acceleration (steps/s) 3")) -> (decimal integer string=w1010:string)  [unwired: 1 in]
            n155 = Number To Fractional String(number=0.0 ("Position (degrees) 3"), precision (6)=i16 0) -> (F-format string=w996:string)  [unwired: 2 in]
            n156 = Number To Decimal String(number=1885 ("Password 4")) -> (decimal integer string=w1001:string)  [unwired: 1 in]
            n157 = Number To Decimal String(number=40000.0 ("Steps/rev 4")) -> (decimal integer string=w1003:string)  [unwired: 1 in]
            n158 = Number To Decimal String(number=4000.0 ("Velocity (steps/s) 3")) -> (decimal integer string=w1007:string)  [unwired: 1 in]
            n159 = Number To Decimal String(number=30003.0 ("Number of Bounces 2")) -> (decimal integer string=w1005:string)  [unwired: 1 in]
            n160 = Concatenate Strings("<", w1010, ",", w996, ",", w1007, ",", w1005, ",", w1003, ",", w1001, ">") -> (w999:string)
            n161 = VISA Write(VISA resource name=w994, write buffer=w999, error in (no error)=w993) -> (VISA resource name out=w992:refnum<visa-resource-name>, error out=w991:errorcluster)  [unwired: 1 out]
          }
        }
      }
      frame True {
        (unwired) ","
        n162 = Number To Decimal String(number=2001.0 ("Acceleration (steps/s) 2")) -> (decimal integer string=w1035:string)  [unwired: 1 in]
        n163 = Number To Fractional String(number=0.0 ("Position (degrees) 2"), precision (6)=i16 2) -> (F-format string=w1021:string)  [unwired: 2 in]
        n164 = Number To Decimal String(number=1885 ("Password 3")) -> (decimal integer string=w1026:string)  [unwired: 1 in]
        n165 = Number To Decimal String(number=400.0 ("Steps/rev 3")) -> (decimal integer string=w1028:string)  [unwired: 1 in]
        n166 = Number To Decimal String(number=5000.0 ("Velocity (steps/s) 2")) -> (decimal integer string=w1032:string)  [unwired: 1 in]
        n167 = Number To Decimal String(number=30002.0 ("Number of Bounces 2")) -> (decimal integer string=w1030:string)  [unwired: 1 in]
        n168 = Concatenate Strings("<", w1035, ",", w1021, ",", w1032, ",", w1030, ",", w1028, ",", w1026, ">") -> (w1024:string)
        n169 = VISA Write(VISA resource name=w1019, write buffer=w1024, error in (no error)=w1018) -> (VISA resource name out=w1017:refnum<visa-resource-name>, error out=w1016:errorcluster)  [unwired: 1 out]
      }
    }
    n170 = VISA Read(VISA resource name=w156, byte count=u32 2500 ("Read Count"), error in (no error)=w157) -> (VISA resource name out=w146:refnum<visa-resource-name>, read buffer=w140:string, error out=w147:errorcluster)  [unwired: 1 out]
    n171 = xnode "Match Regular Expression"("input string"=w140, "regular expression"=w163) -> ("whole match"=→"whole match 2":string, "submatch 2"=w136:string)  [unwired: 4 in, 5 out]
    "Motion Status" <- w136
    n172 = xnode "Match Regular Expression"("input string"=w140, "regular expression"=w145) -> ("whole match"=→"whole match 3":string, "submatch 2"=→"Controller Time":string)  [unwired: 4 in, 5 out]
    n173 = xnode "Match Regular Expression"("input string"=w140, "regular expression"=w160) -> ("whole match"=→"whole match":string, "submatch 2"=w161:string)  [unwired: 4 in, 5 out]
    n174 = Decimal String To Number(string=w161) -> (number=w98:i32)  [unwired: 2 in, 1 out]
    n175 = xnode "Formula"("StepperCurrentPos"=w98) -> ("Result"=w108:dbl)  [unwired: 1 in, 1 out]
    n176 = xnode "Formula"("StepperCurrentPos"=w98) -> ("Result"=w97:dbl)  [unwired: 1 in, 1 out]
    n177 = Number To Fractional String(number=w108, precision (6)=i16 1) -> (F-format string=w106:string)  [unwired: 2 in]
    n178 = Fract/Exp String To Number(string=w106) -> (number=w105:dbl)  [unwired: 3 in, 1 out]
    "Position\n(relative to zeroed position)" <- w105
    n179 = Build Array(w105) -> (w103:dbl[])
    n180 = call "Convert to Dynamic Data"("Array"=w103) -> ("Dynamic Data Type"=w118:dynamicdata)  [unwired: 3 in]
    n181 = xnode "Formula"("Forces"=w81, "Pos"=w118) -> ("Result"=w104:dynamicdata)  [unwired: 1 in, 1 out]
    n182 = xnode ("Set Dynamic Data Attributes")("Signals In"=w104, "Signal Name"="Angle (deg)") -> ("Signals Out"=w116:dynamicdata)  [unwired: 2 in, 1 out]
    n183 = xnode "Formula"("Fx"=w83, "Fy"=w80, "Angle"=w103) -> ("Result"=w102:dbl[])  [unwired: 1 in, 1 out]
    n184 = xnode "Formula"("Fx"=w83, "Fy"=w80, "Angle"=w103) -> ("Result"=w101:dbl[])  [unwired: 1 in, 1 out]
    n185 = feedback-in #1(w97) -> ()
    n186 = Merge Signals(w116, w115, w114, w75, w74) -> (w117:dynamicdata)
    n187 = To Double Precision Float(number=w102) -> (double precision float=w100:dbl[])
    n188 = Index Array(array=w101) -> (element=w73:dbl)  [unwired: 1 in]
    "Lift (N)" <- w73
    n189 = Index Array(array=w100) -> (element=w72:dbl)  [unwired: 1 in]
    "Drag (N)" <- w72
    n190 = Bundle(w73, w72) -> (→"Transformed Lift and Drag Data":cluster{dbl, dbl})  [unwired: 1 in]
    n191 = Equal?(x=w136, y=" LOGGING") -> (x = y?=w109:bool)
    n192 = case shown="True" w109 {
      tunnel: w117 -> [_ w498]
      tunnel: w85 -> [_ w497]
      frame False {
      }
      frame True {
        n193 = call "Write To Measurement File"("Signals"=w498, "Filename"=w497) -> ()  [unwired: 15 in, 3 out]
      }
    }
  }
  n194 = VISA Flush I/O Buffer(VISA resource name=w34, error in (no error)=w33) -> (VISA resource name out=w32:refnum<visa-resource-name>, error out=w31:errorcluster)  [unwired: 1 in]
  n195 = call <vilib>:"DAQmx Clear Task.vi"("task in"=w5, "error in"=w4) -> ()  [unwired: 13 in, 1 out]
  n196 = VISA Close(VISA resource name=w32, error in (no error)=w31) -> (error out=w44:errorcluster)
  n197 = call <vilib>:"Simple Error Handler.vi"("error in (no error)"=w44) -> ()  [unwired: 1 in, 8 out]
